vi "Tranform_to_Lines.vi"(4 "Angle Canceling Resolution":i32=20, 5 "Xintercept Pixel Resolution":dbl, 6 "X Intercept Canceling Resolution":i32=50, 7 "X Size":i32, 8 "Transformed Array":i32[][](array[numeric])) -> (0 "Angle 1":i32, 1 "X Intercept 1":i32, 2 "Angle 2":i32, 3 "X Intercept 2":i32)   [LabVIEW 2009]
panel:
  out "Intensity Graph - For Debugging":i32[][](graph)
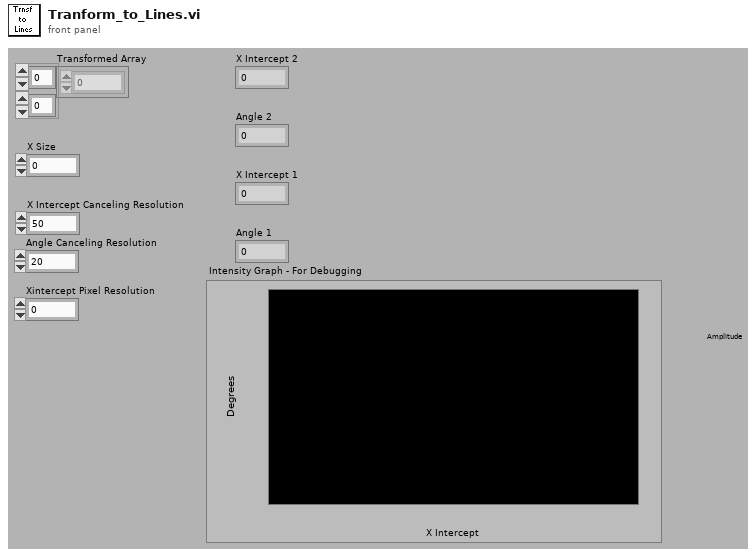
[diagram p1: front panel]
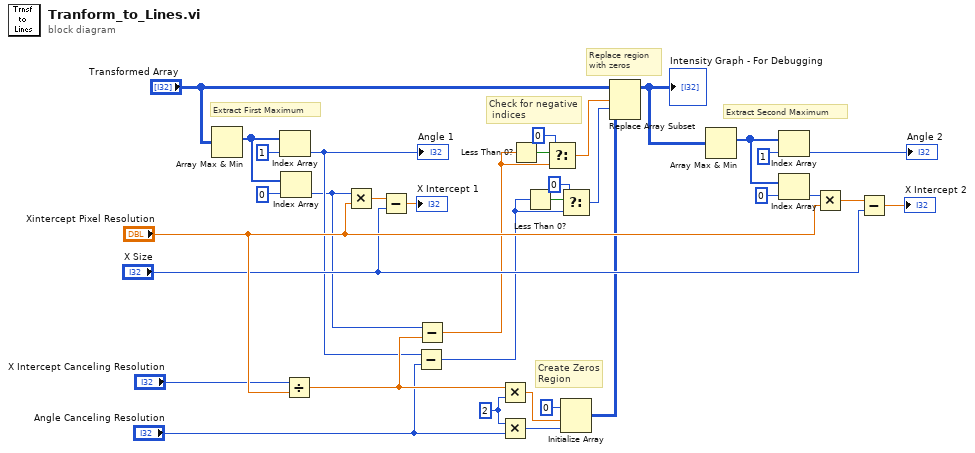
[diagram p0: block diagram]
diagram:
  w21 = 2 ("y")
  # "Create Zeros\nRegion"
  # "Extract Second Maximum"
  # "Replace region\nwith zeros"
  # "Check for negative\n indices"
  # "Extract First Maximum"
  n1 = Array Max & Min(array="Transformed Array") -> (max index (indices)=w12:i32[])  [unwired: 3 out]
  n2 = Index Array(array=w12, index=1) -> (element=w19:i32)
  "Angle 1" <- w19
  n3 = Index Array(array=w12, index=0) -> (element=w18:i32)
  n4 = Divide(x="X Intercept Canceling Resolution", y="Xintercept Pixel Resolution") -> (x/y=w34:dbl)
  n5 = Multiply(x=w18, y="Xintercept Pixel Resolution") -> (x*y=w16:dbl)
  n6 = Subtract(x=w16, y="X Size") -> (x-y=→"X Intercept 1":dbl)
  n7 = Subtract(x=w19, y="Angle Canceling Resolution") -> (x-y=w2:i32)
  n8 = Subtract(x=w18, y=w34) -> (x-y=w6:dbl)
  n9 = Multiply(x=w34, y=w21) -> (x*y=w22:dbl)
  n10 = Multiply(x=w21, y="Angle Canceling Resolution") -> (x*y=w20:i32)
  n11 = Less Than 0?(x=w6) -> (x < 0?=w9:bool)
  n12 = Less Than 0?(x=w2) -> (x < 0?=w4:bool)
  n13 = Select(t=0, s=w9, f=w6) -> (s? t:f=w7:dbl)
  n14 = Select(t=0, s=w4, f=w2) -> (s? t:f=w1:i32)
  n15 = Initialize Array(0 ("element"), w22, w20) -> (w5:i32[][])
  n16 = Replace Array Subset(array="Transformed Array", new element=w5, index (row)=w7, index (col)=w1) -> (w10:i32[][])
  "Intensity Graph - For Debugging" <- w10
  n17 = Array Max & Min(array=w10) -> (max index (indices)=w28:i32[])  [unwired: 3 out]
  n18 = Index Array(array=w28, index=1) -> (element=→"Angle 2":i32)
  n19 = Index Array(array=w28, index=0) -> (element=w27:i32)
  n20 = Multiply(x=w27, y="Xintercept Pixel Resolution") -> (x*y=w25:dbl)
  n21 = Subtract(x=w25, y="X Size") -> (x-y=→"X Intercept 2":dbl)
